vi "Notifier Names.vi"(10 "TimingEngine":T1, 11 "Chassis Name":string) -> (2 "Scalar Notifier":string, 3 "Wfm Notifier":string)   [LabVIEW 2012]
uses:
  Controls/TE_Designator.ctl
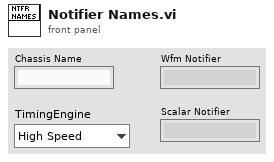
[diagram p1: front panel]
types:
  T1 = typedef "TE_Designator.ctl" = enum16{"High Speed", "Low Speed"}
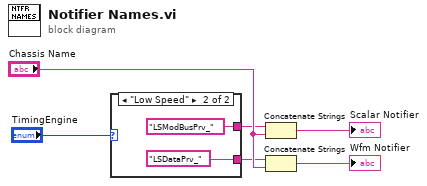
[diagram p0: block diagram]
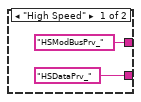
[diagram p2: hidden frame]
diagram:
  n1 = case shown="\"Low Speed\"" "TimingEngine" {
    tunnel: ["HSModBusPrv_" "LSModBusPrv_"] -> w1
    tunnel: ["HSDataPrv_" "LSDataPrv_"] -> w2
    frame "High Speed" {
    }
    frame "Low Speed" {
    }
  }
  n2 = Concatenate Strings(w1, "Chassis Name") -> (→"Scalar Notifier":string)
  n3 = Concatenate Strings(w2, "Chassis Name") -> (→"Wfm Notifier":string)
